vi "cDAQ_VI_Leo_Modified.vi"() -> ()   [LabVIEW 2022 SP3]
uses:
  <vilib>/Analysis/baseanly.llb/Mean (DBL).vi
  STOP_GLOBAL.vi
  <vilib>/addons/control/pid/pid.llb/PID EGU to Percentage (DBL).vi
  <vilib>/DAQmx/miscellaneous.llb/DAQmx Fill In Error Info.vi
  <vilib>/DAQmx/configure/timing.llb/DAQmx Timing (Sample Clock).vi
  <vilib>/DAQmx/read.llb/DAQmx Read (Analog 1D Wfm NChan NSamp).vi
  <vilib>/Analysis/NI_AALBase.lvlib
  <vilib>/addons/control/pid/NI_PID_pid.lvlib
  <vilib>/addons/control/pid/NI_PID_autopid.lvlib
panel:
  in  "Tab Control":enum32{"Manual", "Automatic"}(tab)
  in  "Channel Array":dbl[](array[slide]) scale=-9.0..5.067
  out "error out 5":errorcluster
  out "Output":dbl(slide) scale=0.0..5.067
  in  "PID gains":T1={"proportional gain (Kc)"=1.0, "integral time (Ti, min)"=0.01, "derivative time (Td, min)"=0.0} {"derivative time (Td, min)" format="%.7f"; "integral time (Ti, min)" format="%.7f"; "proportional gain (Kc)" format="%.3f"}
  out "elapsed time (s)":dbl format="%.3f"
  in  "setpoint profile":cluster{"time (s)":dbl, "setpoint":dbl}[](array[cluster]) {"setpoint" format="%.2f"; "time (s)" format="%.3f"}
  in  "reinitialize? (F)":bool
  in  "autotune? (F)":bool
  out "Waveform Chart 2":cluster{"setpoint":dbl, dbl}(graph) caption="Waveform Chart"
  out "XY Graph":cluster{dbl[], dbl[]}[](graph)
  out "error out":errorcluster
  out "All Channel Graph":cluster{dbl[], dbl[]}[](graph)
  out "Thrust":cluster{dbl[], dbl[]}(graph)
  out "Chamber Pressure":cluster{dbl[], dbl[]}(graph)
  out "Supply Pressure":cluster{dbl[], dbl[]}(graph)
  out "MassFlow":cluster{dbl[], dbl[]}(graph)
  out "Temperature":cluster{dbl[], dbl[]}(graph)
  out "error out 3":errorcluster caption="error out"
  out "error out 2":errorcluster
  in  "rate":dbl=1000.0 format="%0.2f"
  in  "number of samples":i32=100
  in  "File Format":string
  in  "File Name Out":string
  in  "Data Collection Folder":path
  out "Temperature":dynamicdata(graph)
  out "Numeric 2":i32
  out "Thrust lb":dynamicdata(graph)
  in  "Types of Testing":enum32{"Test Firing", "Cold Flow Rig"}(tab)
  out "Saving Data":bool
  out "Filename Out":path
  in  "Collect Data?":bool=TRUE caption="Enable"
  in  "Collect Data? 2":bool=TRUE caption="Enable"
  out "Saving Data":bool
  out "Filename Out":path
  out "Supply Pressure PSI":dynamicdata(graph)
  out "1st channel NI 9252":dynamicdata(graph)
  out "Mass Flow L/min":dynamicdata(graph)
  out "Chamber Pressure PSI":dynamicdata(graph)
  # "Control Loop"
  # "DATA LOGGING INFORMATION"
  # "ANALOG VOLTAGE OUTPUT"
  # "RESULTS"
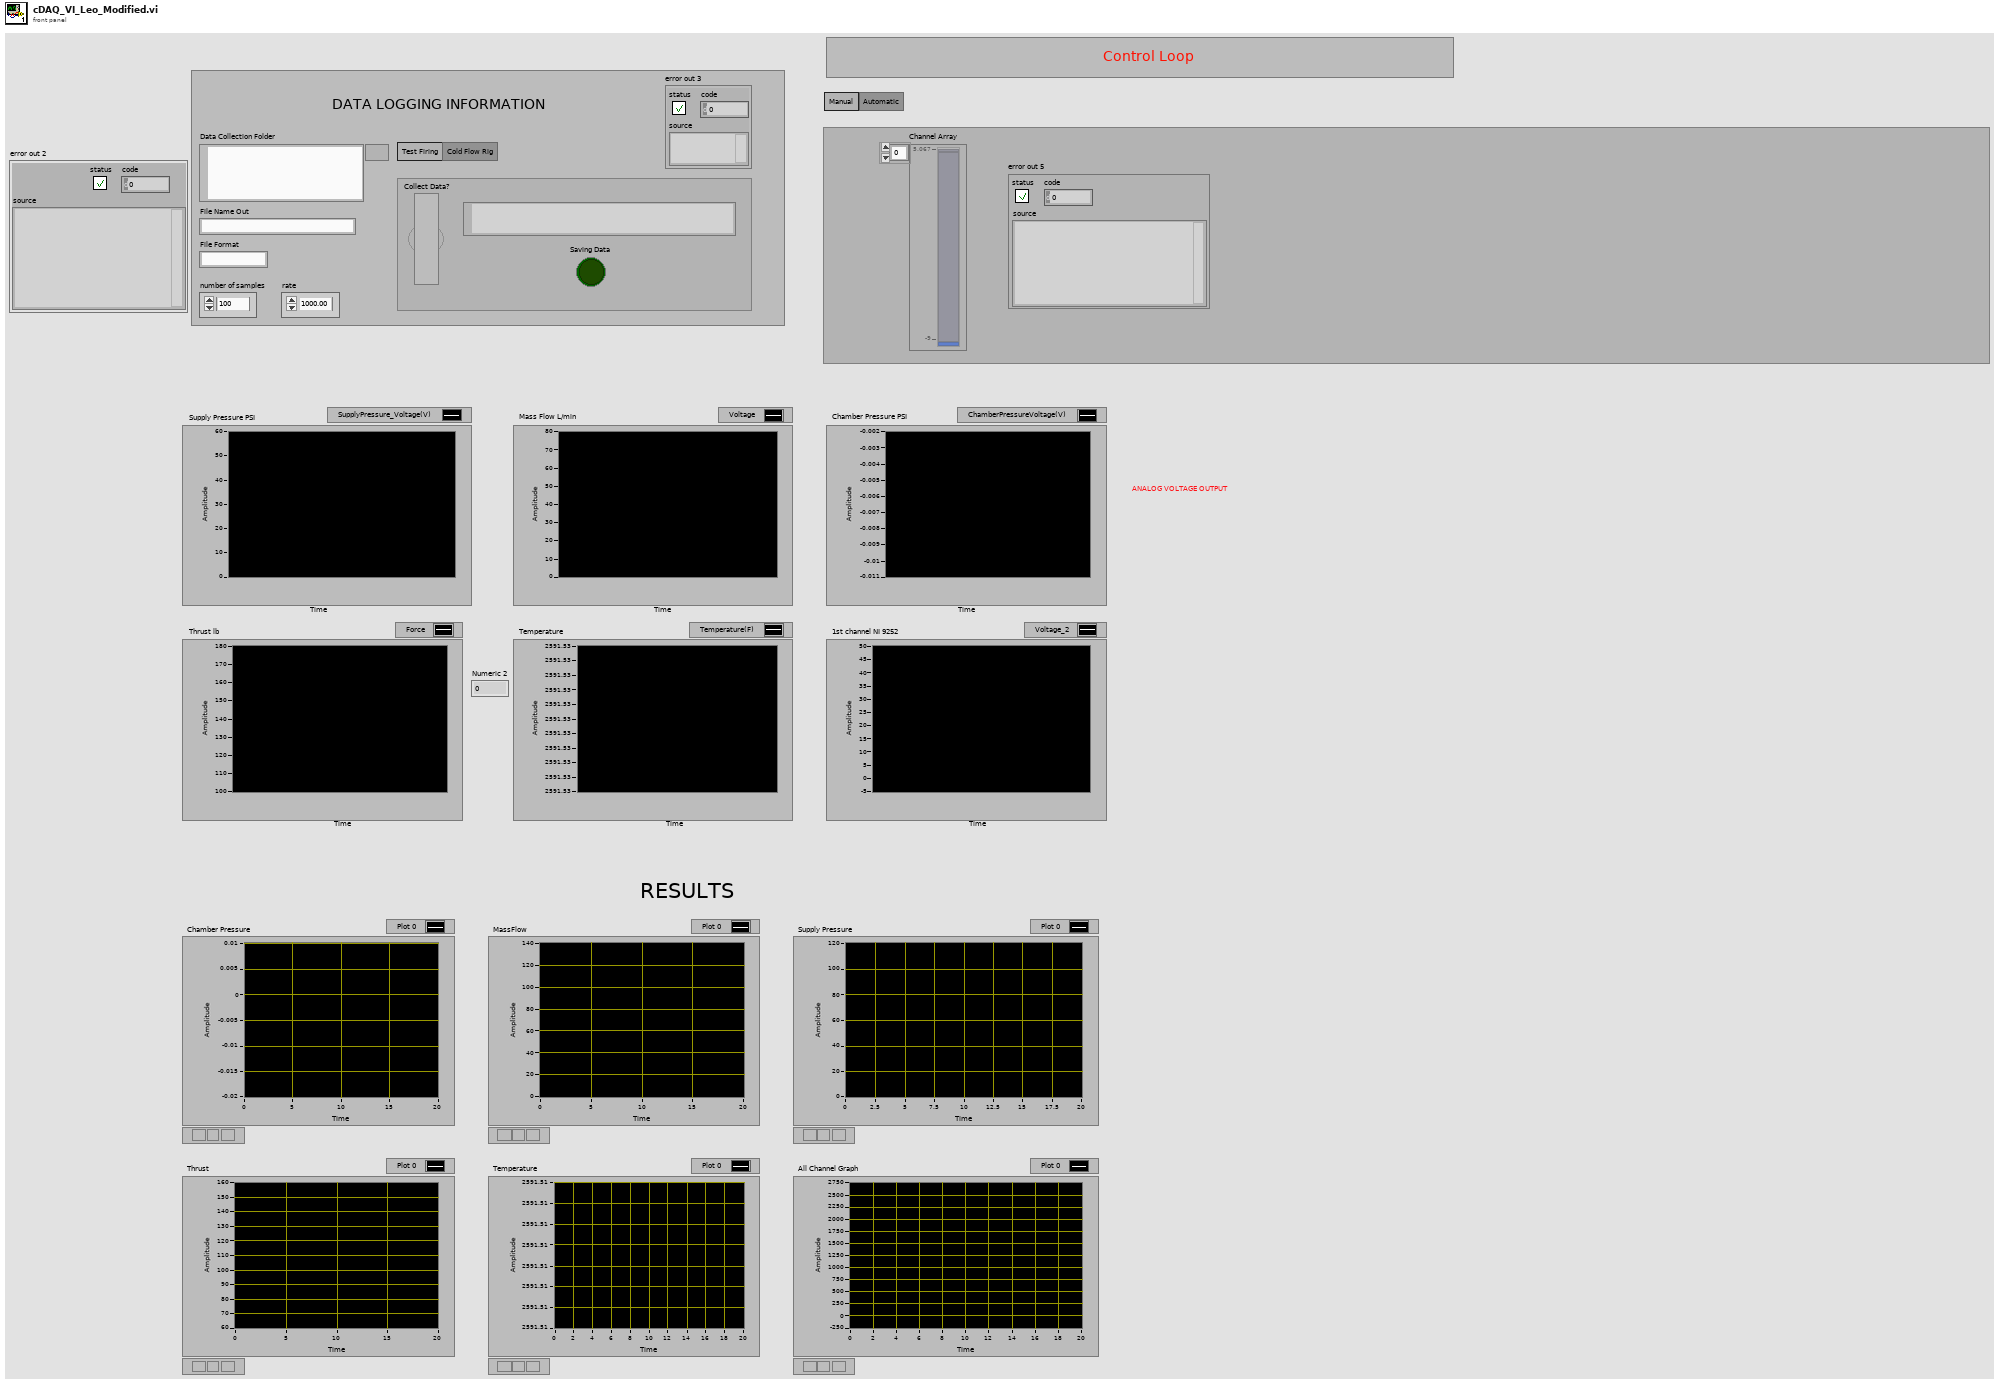
[diagram p1: front panel]
types:
  T1 = cluster{"proportional gain (Kc)":dbl, "integral time (Ti, min)":dbl, "derivative time (Td, min)":dbl}
  T2 = cluster{"controller type":u16, "relay cycles":i32, "relay amplitude":dbl, "control specification":u16, "PV noise level":dbl}
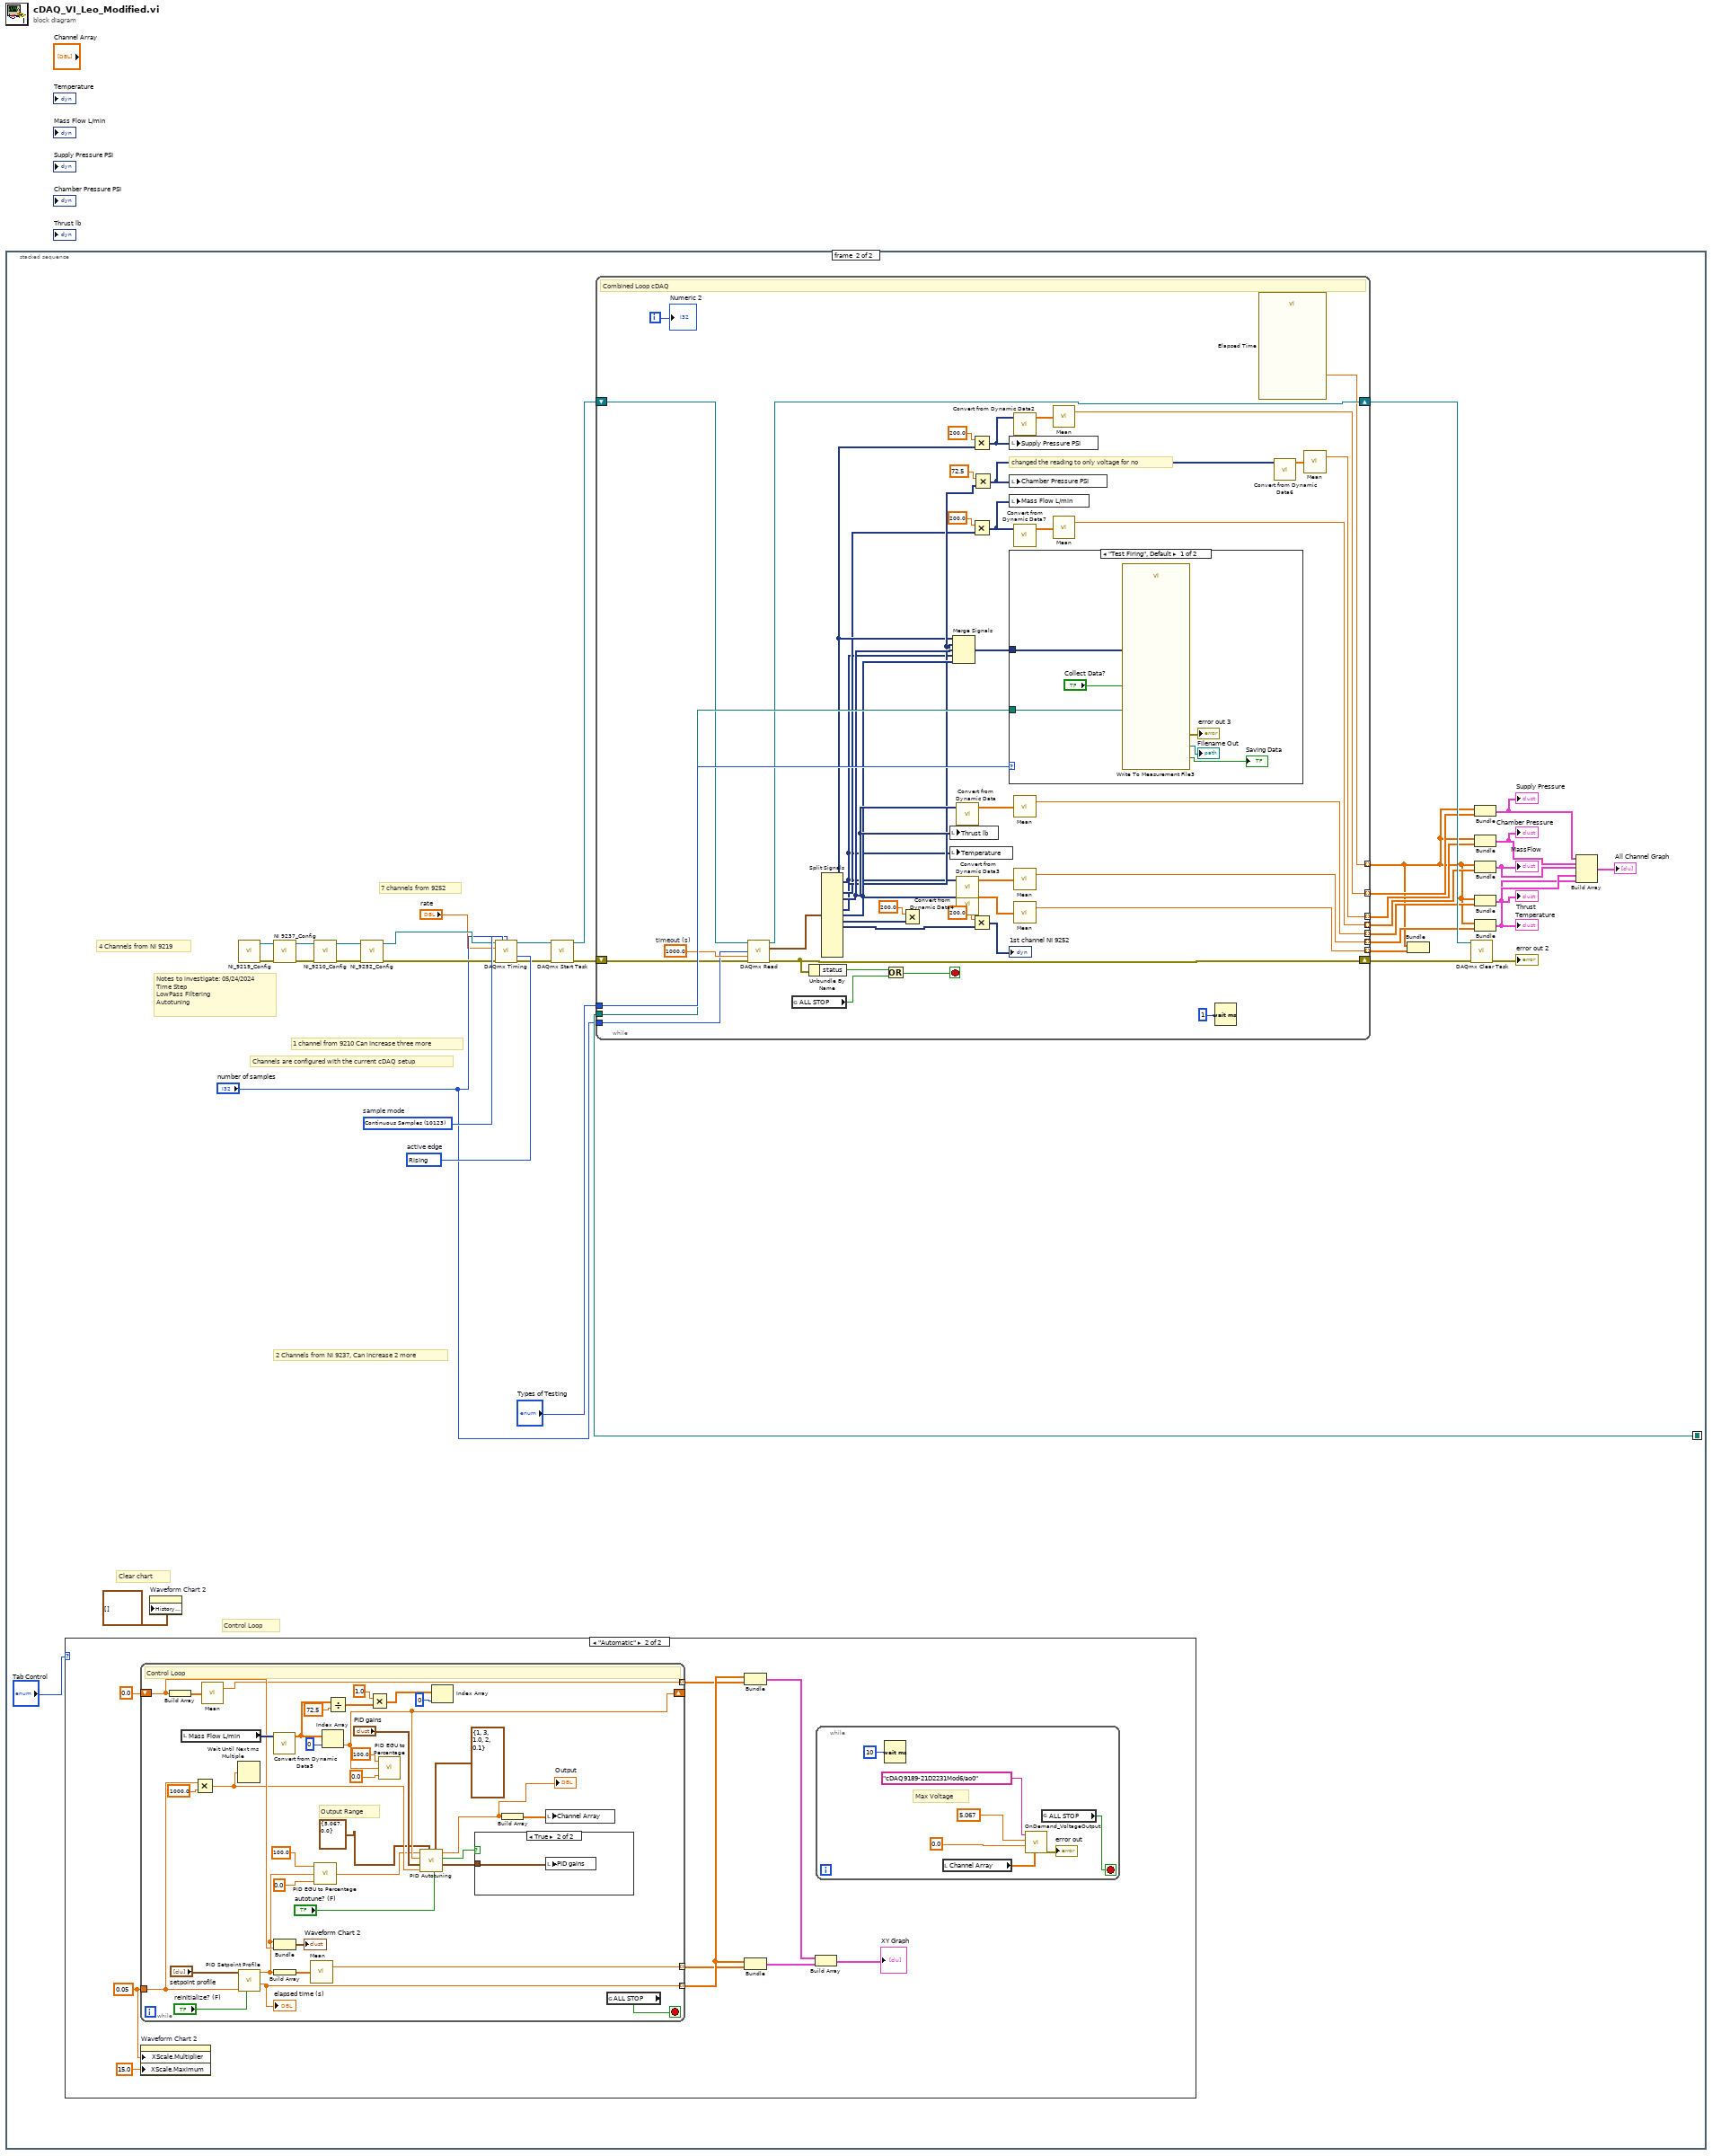
[diagram p0: block diagram]
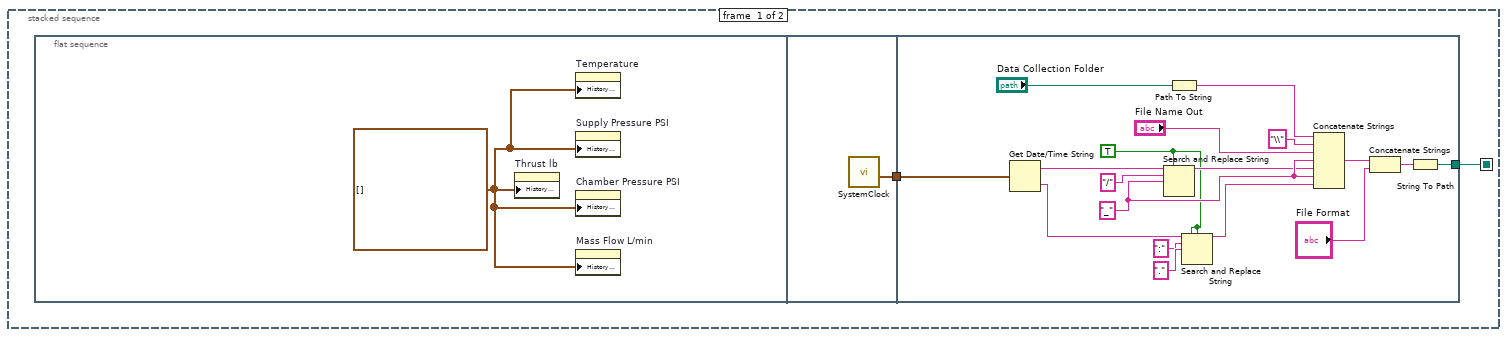
[diagram p2: hidden frame]
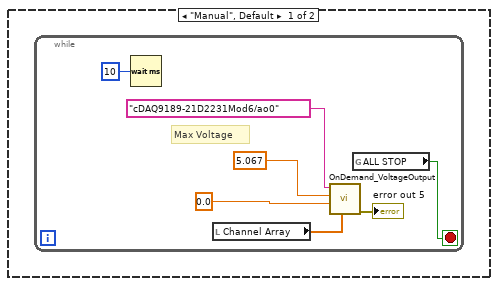
[diagram p3: hidden frame]
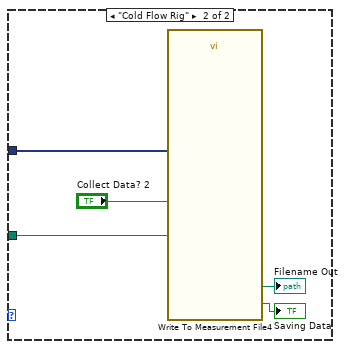
[diagram p5: hidden frame]
diagram:
  n1 = stacked-sequence {
    seq-local: [w1 _] -> [_ w57]
    frame #0 {
      n2 = flat-sequence {
        tunnel: [w4] -> w2
        tunnel: w2 -> [w11]
        tunnel: [w10] -> w1
        frame #0 {
          w3 = waveform(dbl)[] []
          n3 = property on="Thrust lb" class="WFChart (strict)"("History Data"=w3) -> ()  [unwired: 2 in, 2 out]
          n4 = property on="Temperature" class="WFChart (strict)"("History Data"=w3) -> ()  [unwired: 2 in, 2 out]
          n5 = property on="Supply Pressure PSI" class="WFChart (strict)"("History Data"=w3) -> ()  [unwired: 2 in, 2 out]
          n6 = property on="Chamber Pressure PSI" class="WFChart (strict)"("History Data"=w3) -> ()  [unwired: 2 in, 2 out]
          n7 = property on="Mass Flow L/min" class="WFChart (strict)"("History Data"=w3) -> ()  [unwired: 2 in, 2 out]
        }
        frame #1 {
          n8 = call "SystemClock.vi"() -> ("LabVIEW Time Stamp"=w4:timestamp)  [unwired: 9 in, 2 out]
        }
        frame #2 {
          w6 = TRUE ("replace all? (F)")
          w19 = "_" ("string")
          n9 = Get Date/Time String(seconds (now)=w11) -> (date string=w13:string, time string=w16:string)  [unwired: 2 in]
          n10 = Search and Replace String(replace all?=w6, input string=w13, search string="/", replace string=w19) -> (result string=w15:string)  [unwired: 4 in, 3 out]
          n11 = Path To String(path="Data Collection Folder") -> (string=w8:string)
          n12 = Search and Replace String(replace all?=w6, case sensitive?=w6, input string=w16, search string=":", replace string="." ("replace string (\"\")")) -> (result string=w20:string)  [unwired: 3 in, 3 out]
          n13 = Concatenate Strings(w8, "\\" ("string"), "File Name Out", w19, w15, w19, w20) -> (w21:string)
          n14 = Concatenate Strings(w21, "File Format") -> (w22:string)
          n15 = String To Path(string=w22) -> (path=w10:path)
        }
      }
    }
    frame #1 {
      w55 = 10123 items=["Finite Samples"=10178, "Continuous Samples"=10123, "Hardware Timed Single Point"=12522]  # sample mode
      w56 = 10280 items=["Rising"=10280, "Falling"=10171]  # active edge
      # "Control Loop"
      # "Clear chart"
      # "Notes to investigate: 05/24/2024\nTime Step\nLowPass FIltering\nAutotuning"
      # "Channels are configured with the current cDAQ setup"
      # "7 channels from 9252"
      # "1 channel from 9210 Can Increase three more"
      # "2 Channels from NI 9237, Can increase 2 more"
      # "4 Channels from NI 9219"
      n16 = case shown="\"Automatic\"" "Tab Control" {
        frame "Manual", Default {
          n17 = while {
            stop <- w65 stop-if-true
            # "Max Voltage"
            n18 = Wait (ms)(milliseconds to wait=u32 10) -> ()  [unwired: 1 out]
            n19 = local read "Channel Array"() -> (w61:dbl[])
            n20 = call "OnDemand_VoltageOutput.vi"("Channel Array"=w61, "minimum voltage"=0.0, "maximum voltage"=5.067, "physical channels"="cDAQ9189-21D2231Mod6/ao0") -> ("error out"=→"error out 5":errorcluster)  [unwired: 7 in]
            n21 = global read "STOP_GLOBAL.vi" "ALL STOP"() -> (w65:bool)
          }
        }
        frame "Automatic" {
          w74 = 0.05 ("dt (s)")
          n22 = while {
            shift-right: [w85] -> _
            shift-left: 0.0 -> [w99]
            tunnel: w74 -> [w102]
            tunnel: [w100] -> w69 mode=indexing
            tunnel: [w98] -> w67 mode=indexing
            tunnel: [w94] -> w68 mode=indexing
            stop <- w117 stop-if-true
            # "Output Range"
            # "Control Loop"
            n23 = Build Array(w99) -> (w97:dbl[])
            n24 = local read "Mass Flow L/min"() -> (w116:dynamicdata)
            n25 = Multiply(x=w102, y=1000.0) -> (x*y=w90:dbl)
            n26 = call-poly <vilib>:"Mean.vi"("X"=w97) -> ("mean"=w98:dbl)  [unwired: 1 out]
            n27 = Wait Until Next ms Multiple(millisecond multiple=w90) -> ()  [unwired: 1 out]
            n28 = call <vilib>:"PID Setpoint Profile.vi"("reinitialize? (F)"="reinitialize? (F)", "dt (s)"=w102, "setpoint profile"="setpoint profile") -> ("elapsed time (s)"=w100:dbl, "setpoint"=w96:dbl)  [unwired: 3 in, 2 out]
            "elapsed time (s)" <- w100
            n29 = call "Convert from Dynamic Data5"("Dynamic Data Type"=w116) -> ("Array"=w111:dbl[])  [unwired: 3 in]
            n30 = Bundle("setpoint"=w96, w99) -> (→"Waveform Chart 2":cluster{"setpoint":dbl, dbl})  [unwired: 1 in]
            n31 = Build Array(w96) -> (w95:dbl[])
            n32 = call-poly <vilib>:"Mean.vi"("X"=w95) -> ("mean"=w94:dbl)  [unwired: 1 out]
            n33 = call-poly <vilib>:"PID EGU to Percentage.vi"("minimum (EGU)"=0.0, "input (EGU)"=w96, "maximum (EGU)"=100.0) -> ("% span"=w84:dbl)
            n34 = Index Array(array=w111, index=0) -> (element=w85:dbl)
            n35 = Divide(x=w111, y=72.5 ("x")) -> (x/y=w114:dbl[])
            n36 = Multiply(x=1.0, y=w114) -> (x*y=w113:dbl[])
            n37 = call-poly <vilib>:"PID EGU to Percentage.vi"("minimum (EGU)"=0.0, "input (EGU)"=w85, "maximum (EGU)"=100.0) -> ()  [unwired: 1 out]
            n38 = call <vilib>:"PID Autotuning.vi"("autotune? (F)"="autotune? (F)", "autotuning parameters"=T2 {"controller type"=1, "relay cycles"=3, "relay amplitude"=1.0, "control specification"=2, "PV noise level"=0.1}, "output range"=cluster{"output high":dbl, "output low":dbl} {"output high"=5.067, "output low"=0.0}, "dt (s)"=w90, "PID gains"="PID gains", "process variable"=w85, "setpoint"=w84) -> ("PID gains out"=w88:T1, "tuning completed?"=w87:bool, "output"=w82:dbl)  [unwired: 1 in, 1 out]
            "Output" <- w82
            n39 = Index Array(array=w113, index=0) -> ()  [unwired: 1 out]
            n40 = case shown="True" w87 {
              tunnel: w88 -> [_ w118]
              frame False {
              }
              frame True {
                n41 = local write "PID gains"(w118) -> ()
              }
            }
            n42 = Build Array(w82) -> (w101:dbl[])
            n43 = local write "Channel Array"(w101) -> ()
            n44 = global read "STOP_GLOBAL.vi" "ALL STOP"() -> (w117:bool)
          }
          n45 = property on="Waveform Chart 2" class="WFChart (strict)"("XScale.Multiplier"=w74, "XScale.Maximum"=15.0 ("X Scale.Range:Maximum")) -> ()  [unwired: 2 in, 2 out]
          n46 = Bundle(w69, w67) -> (w70:cluster{dbl[], dbl[]})  [unwired: 1 in]
          n47 = Bundle(w69, w68) -> (w71:cluster{dbl[], dbl[]})  [unwired: 1 in]
          n48 = Build Array(w70, w71) -> (→"XY Graph":cluster{dbl[], dbl[]}[])
          n49 = while {
            stop <- w81 stop-if-true
            # "Max Voltage"
            n50 = Wait (ms)(milliseconds to wait=u32 10) -> ()  [unwired: 1 out]
            n51 = local read "Channel Array"() -> (w77:dbl[])
            n52 = call "OnDemand_VoltageOutput.vi"("Channel Array"=w77, "minimum voltage"=0.0, "maximum voltage"=5.067, "physical channels"="cDAQ9189-21D2231Mod6/ao0") -> ("error out"=→"error out":errorcluster)  [unwired: 7 in]
            n53 = global read "STOP_GLOBAL.vi" "ALL STOP"() -> (w81:bool)
          }
        }
      }
      n54 = property on="Waveform Chart 2" class="WFChart (strict)"("History Data"=cluster{"setpoint":dbl, dbl}[] []) -> ()  [unwired: 2 in, 2 out]
      n55 = call "NI_9219_Config.vi"() -> ("error out"=w37:errorcluster, "task out"=w48:refnum<k21>)  [unwired: 10 in]
      n56 = call "NI 9237_Config.vi"("error in"=w37, "task in"=w48) -> ("error out"=w46:errorcluster, "task out"=w47:refnum<k21>)  [unwired: 8 in]
      n57 = call "NI_9210_Config.vi"("error in"=w46, "task in"=w47) -> ("error out"=w44:errorcluster, "task out"=w45:refnum<k21>)  [unwired: 8 in]
      n58 = call "NI_9252_Config.vi"("error in"=w44, "task in"=w45) -> ("error out"=w42:errorcluster, "task out"=w43:refnum<k21>)  [unwired: 8 in]
      n59 = call-poly <vilib>:"DAQmx Timing.vi"("task/channels in"=w43, "sample mode"=w55, "samples per channel"="number of samples", "rate"="rate", "active edge"=w56, "error in"=w42) -> ("task out"=w54:refnum<k21>, "error out"=w53:errorcluster)  [unwired: 8 in]
      n60 = call <vilib>:"DAQmx Start Task.vi"("task/channels in"=w54, "error in"=w53) -> ("task out"=w52:refnum<k21>, "error out"=w51:errorcluster)  [unwired: 12 in]
      n61 = while {
        tunnel: "Types of Testing" -> [w162]
        tunnel: [w160] -> w32 mode=indexing
        tunnel: w57 -> [w155]
        tunnel: "number of samples" -> [w153]
        shift-right: [w149] -> w49
        shift-left: w51 -> [w152]
        shift-right: [w150] -> w50
        shift-left: w52 -> [w151]
        tunnel: [w145] -> w34 mode=indexing
        tunnel: [w142] -> w33 mode=indexing
        tunnel: [w140] -> w35 mode=indexing
        tunnel: [w126] -> w36 mode=indexing
        tunnel: [w133] -> w38 mode=indexing
        tunnel: [w119] -> w31 mode=indexing
        i -> [w163]
        stop <- w156 stop-if-true
        w158 = 1000.0  # timeout (s)
        # "changed the reading to only voltage for no"
        # "Combined Loop cDAQ"
        n62 = call-poly <vilib>:"DAQmx Read.vi"("task/channels in"=w151, "number of samples per channel"=w153, "timeout"=w158, "error in"=w152) -> ("task out"=w150:refnum<k21>, "data"=w154:waveform(dbl)[], "error out"=w149:errorcluster)  [unwired: 9 in]
        n63 = global read "STOP_GLOBAL.vi" "ALL STOP"() -> (w157:bool)
        n64 = Unbundle By Name(w149) -> ("status"=w159:bool)
        n65 = Split Signals(w154) -> (w129:dynamicdata, w130:dynamicdata, w127:dynamicdata, w137:dynamicdata, w125:dynamicdata, w135:dynamicdata, w123:dynamicdata, w121:dynamicdata)  [unwired: 15 in, 7 out]
        n66 = Or(x=w159, y=w157) -> (x .or. y?=w156:bool)
        n67 = Multiply(x=200.0, y=w123) -> ()  [unwired: 1 out]
        n68 = local write "Thrust lb"(w137) -> ()
        n69 = local write "Temperature"(w125) -> ()
        n70 = Merge Signals(w129, w130, w137, w125, w135) -> (w139:dynamicdata)
        n71 = call "Convert from Dynamic Data"("Dynamic Data Type"=w137) -> ("Array"=w161:dbl[])  [unwired: 3 in]
        n72 = call "Convert from Dynamic Data3"("Dynamic Data Type"=w125) -> ("Array"=w138:dbl[])  [unwired: 3 in]
        n73 = call "Convert from Dynamic Data4"("Dynamic Data Type"=w135) -> ("Array"=w134:dbl[])  [unwired: 3 in]
        n74 = Multiply(x=200.0, y=w129) -> (x*y=w132:dynamicdata)
        n75 = Multiply(x=200.0, y=w127) -> (x*y=w128:dynamicdata)
        n76 = Multiply(x=200.0, y=w121) -> (x*y=→"1st channel NI 9252":dynamicdata)
        n77 = Multiply(x=72.5, y=w130) -> (x*y=w136:dynamicdata)
        n78 = local write "Supply Pressure PSI"(w132) -> ()
        n79 = local write "Chamber Pressure PSI"(w136) -> ()
        n80 = local write "Mass Flow L/min"(w128) -> ()
        n81 = case shown="\"Test Firing\", Default" w162 {
          tunnel: w155 -> [w167 w171]
          tunnel: w139 -> [w165 w170]
          frame "Test Firing", Default {
            n82 = call "Write To Measurement File3"("Signals"=w165, "Enable"="Collect Data?", "Filename"=w167) -> ("Filename Out"=→"Filename Out":path, "Saving Data"=→"Saving Data":bool, "error out"=→"error out 3":errorcluster)  [unwired: 14 in]
          }
          frame "Cold Flow Rig" {
            n83 = call "Write To Measurement File4"("Signals"=w170, "Enable"="Collect Data? 2", "Filename"=w171) -> ("Filename Out"=→"Filename Out":path, "Saving Data"=→"Saving Data":bool)  [unwired: 14 in, 1 out]
          }
        }
        n84 = call "Convert from Dynamic Data2"("Dynamic Data Type"=w132) -> ("Array"=w144:dbl[])  [unwired: 3 in]
        n85 = call "Convert from Dynamic Data7"("Dynamic Data Type"=w128) -> ("Array"=w141:dbl[])  [unwired: 3 in]
        n86 = call-poly <vilib>:"Mean.vi"("X"=w161) -> ("mean"=w160:dbl)  [unwired: 1 out]
        n87 = call-poly <vilib>:"Mean.vi"("X"=w138) -> ("mean"=w126:dbl)  [unwired: 1 out]
        n88 = call-poly <vilib>:"Mean.vi"("X"=w134) -> ("mean"=w133:dbl)  [unwired: 1 out]
        n89 = call-poly <vilib>:"Mean.vi"("X"=w144) -> ("mean"=w145:dbl)  [unwired: 1 out]
        n90 = call-poly <vilib>:"Mean.vi"("X"=w141) -> ("mean"=w140:dbl)  [unwired: 1 out]
        n91 = Wait (ms)(milliseconds to wait=u32 1) -> ()  [unwired: 1 out]
        n92 = call "Elapsed Time"() -> ("Elapsed Time (s)"=w119:dbl)  [unwired: 12 in, 7 out]
        n93 = call "Convert from Dynamic Data6"("Dynamic Data Type"=w136) -> ("Array"=w143:dbl[])  [unwired: 3 in]
        n94 = call-poly <vilib>:"Mean.vi"("X"=w143) -> ("mean"=w142:dbl)  [unwired: 1 out]
        "Numeric 2" <- w163
      }
      n95 = Bundle(w31, w38) -> ()  [unwired: 1 in, 1 out]
      n96 = call <vilib>:"DAQmx Clear Task.vi"("task in"=w50, "error in"=w49) -> ("error out"=→"error out 2":errorcluster)  [unwired: 13 in]
      n97 = Bundle(w31, w34) -> (w30:cluster{dbl[], dbl[]})  [unwired: 1 in]
      "Supply Pressure" <- w30
      n98 = Bundle(w31, w33) -> (w29:cluster{dbl[], dbl[]})  [unwired: 1 in]
      "Chamber Pressure" <- w29
      n99 = Bundle(w31, w35) -> (w28:cluster{dbl[], dbl[]})  [unwired: 1 in]
      "MassFlow" <- w28
      n100 = Bundle(w31, w32) -> (w27:cluster{dbl[], dbl[]})  [unwired: 1 in]
      "Thrust" <- w27
      n101 = Bundle(w31, w36) -> (w26:cluster{dbl[], dbl[]})  [unwired: 1 in]
      "Temperature" <- w26
      n102 = Build Array(w30, w29, w28, w27, w26) -> (→"All Channel Graph":cluster{dbl[], dbl[]}[])
    }
  }
